vi "callback_lvssh2_userauth_keyboard_interactive_response_function.vi"(8 "error in (no error)":errorcluster, 9 "prompts":T1[](array[typedef]), 10 "instruction":string, 11 "name":string) -> (0 "error out":errorcluster, 2 "responses":string[](array[string]))   [LabVIEW 2017, in "support.lvlib"]
doc: "Called when authenticating with libssh2 using <B>libssh2_userauth_keyboard_interactive</B>.\n\n<B>name</B> name of the user attempting keyboard-interactive authentication.\n<B>instruction</B>\n<B>prompts</B> challenges provided by the server\n\nReturns the response to the challenges."
uses:
  support.lvlib
  libssh2/lvssh2_userauth_keyboard_interactive_prompt.ctl
  libssh2/libssh2.lvlib
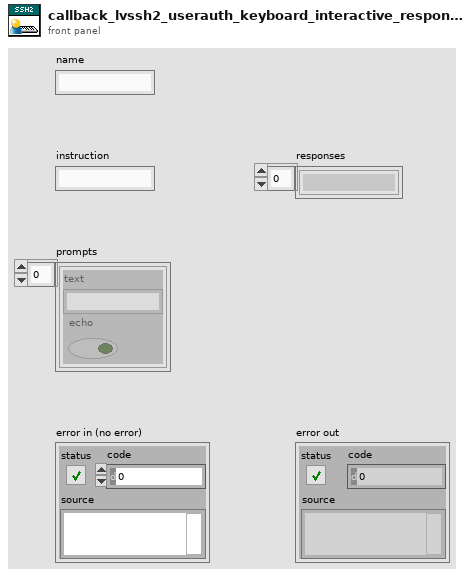
[diagram p1: front panel]
types:
  T1 = typedef "libssh2.lvlib/lvssh2_userauth_keyboard_interactive_prompt.ctl" = cluster{"text":string, "echo":bool}
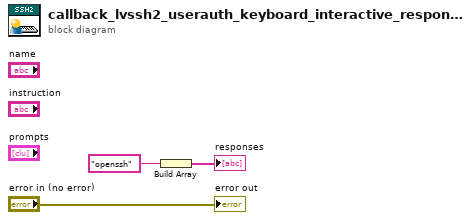
[diagram p0: block diagram]
diagram:
  n1 = Build Array("openssh") -> (→"responses":string[])
  "error out" <- "error in (no error)"
